vi "uTransport_IsValid.vi"(8 "error in (no error)":errorcluster, 11 "uActor in":refnum<class "uActor.lvclass">) -> (0 "error out":errorcluster, 2 "IsValid?":bool, 3 "uActor out":refnum<class "uActor.lvclass">)   [LabVIEW 2023, in "uLib.lvlib" / "uActor.lvclass"]
doc: "Check if the Actor is still Alive."
uses:
  uActor.lvclass
  uActor.lvclass/uActor.ctl
  uTransport/uTransport_uActor/uTransport_uActor.lvclass
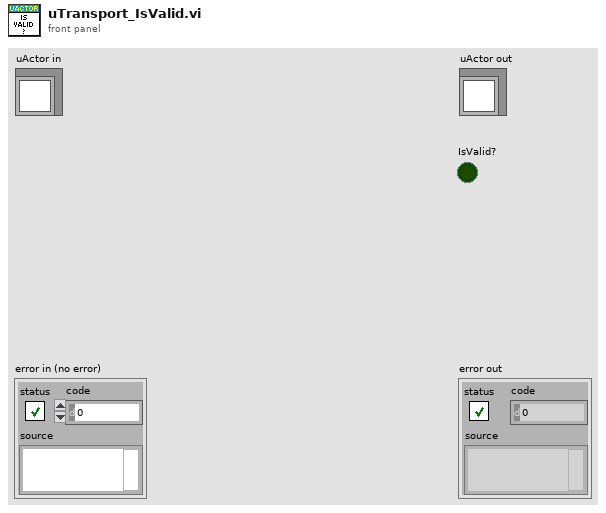
[diagram p1: front panel]
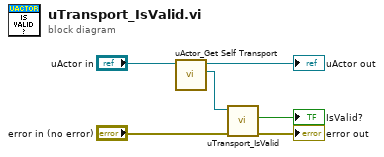
[diagram p0: block diagram]
diagram:
  n1 = call "uActor_Get Self Transport.vi"("uActor in"="uActor in") -> ("Actor Transport"=w6:refnum<class "uTransport_uActor.lvclass">, "uActor out"=→"uActor out":refnum<class "uActor.lvclass">)  [unwired: 9 in]
  n2 = call-dynamic "uTransport_IsValid.vi"("error in (no error)"="error in (no error)", "uTransport_uActor in"=w6) -> ("error out"=→"error out":errorcluster, "IsValid?"=→"IsValid?":bool)  [unwired: 7 in, 1 out]
